vi "Teleop.vi"(10 "Match Info":T1={"Autonomous Elapsed Seconds"=0.0, "TeleOp Elapsed Seconds"=0.0, "Disabled Elapsed Seconds"=0.0, "Visited Autonomous"=FALSE, "Visited TeleOp"=FALSE, "Visited Disabled"=FALSE, "Autonomous Settings"={"Autonomous Style"=enum."Independent", "VI Refnum"=refnum}}, 11 "Call Context":T2) -> ()   [LabVIEW 2015]
doc: "This VI is called for each TeleOp packet received from the DS where the robot is not disabled. It is often used to read from the joysticks and update I/O or to update setpoints for timed control loops. It should complete and return within 20 milliseconds or it may miss DS packets."
uses:
  <vilib>/Rock Robotics/WPI/DriverStation/WPI_DriverStationDerivedRobotMode.ctl
  <vilib>/Rock Robotics/WPI/DriverStation/WPI_DriverStationMatch Info.ctl
  <vilib>/Rock Robotics/WPI/Relay/WPI_RelayValue.ctl
  <vilib>/Rock Robotics/WPI/Utilities/WPI_GetSetVariantRefNum.vi
  <vilib>/Rock Robotics/Network Tables/SD Write Boolean Array.vi
  <vilib>/Rock Robotics/Network Tables/SD Write Numeric Array.vi
  <vilib>/Rock Robotics/Network Tables/SD Read Boolean.vi
  <vilib>/Rock Robotics/Network Tables/SD Read Number.vi
  <vilib>/Rock Robotics/WPI/RobotDrive/WPI_RobotDriveMecanumDrive_Cartesian.vi
panel:
  out "Sample Slider 0":dbl(slide) scale=0.0..5.0
  out "Sample Boolean 1":bool
  out "Sample Boolean 0":bool
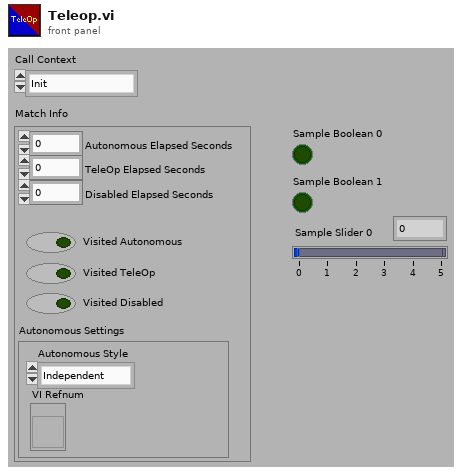
[diagram p1: front panel]
types:
  T1 = typedef "WPI_DriverStationMatch Info.ctl" = cluster{"Autonomous Elapsed Seconds":dbl, "TeleOp Elapsed Seconds":dbl, "Disabled Elapsed Seconds":dbl, "Visited Autonomous":bool, "Visited TeleOp":bool, "Visited Disabled":bool, "Autonomous Settings":cluster{"Autonomous Style":enum16{"Iterative", "Independent"}, "VI Refnum":refnum<vi>}}
  T2 = typedef "WPI_DriverStationDerivedRobotMode.ctl" = enum16{"Init", "Execute", "Stop"}
  T3 = typedef "WPI_RelayValue.ctl" = enum16{"Off", "On", "Forward", "Reverse"}
  T4 = typedef "WPI_JoystickDevRef.ctl" = cluster{"Device":T5}
  T5 = typedef "WPI_JoystickDeviceEnum.ctl" = enum16{"USB 0", "USB 1", "USB 2", "USB 3", "USB 4", "USB 5"}
  T6 = cluster{"Axes[0]":dbl, "Axes[1]":dbl, "Axes[2]":dbl, "Axes[3]":dbl, "Axes[4]":dbl, "Axes[5]":dbl, "Axes[6]":dbl, "Axes[7]":dbl, "Axes[8]":dbl}
  T7 = cluster{"Buttons[0]":bool, "Buttons[1]":bool, "Buttons[2]":bool, "Buttons[3]":bool, "Buttons[4]":bool, "Buttons[5]":bool, "Buttons[6]":bool, "Buttons[7]":bool, "Buttons[8]":bool}
  T8 = typedef "WPI_SwitchDevRef.ctl" = cluster{"DevStatus":errorcluster, "DIO Channel":T9, "CntIndex":T10, "Normally Closed":bool}
  T9 = typedef "FPGA_DIOChannel.ctl" = enum8{"DIO 0", "DIO 1", "DIO 2", "DIO 3", "DIO 4", "DIO 5", "DIO 6", "DIO 7", "DIO 8", "DIO 9", "DIO MXP 0", "DIO MXP 1", "DIO MXP 2", "DIO MXP 3", "DIO MXP 4", "DIO MXP 5", "DIO MXP 6", "DIO MXP 7", "DIO MXP 8", "DIO MXP 9", "DIO MXP 10", "DIO MXP 11", "DIO MXP 12", "DIO MXP 13", "DIO MXP 14", "DIO MXP 15", "Invalid"}
  T10 = typedef "FPGA_CounterCtrSystemIndex.ctl" = enum8{"Ctr 0", "Ctr 1", "Ctr 2", "Ctr 3", "Ctr 4", "Ctr 5", "Ctr 6", "Ctr 7", "Invalid"}
  T11 = typedef "WPI_RobotDriveDevRef.ctl" = cluster{"DevStatus":errorcluster, "Motors[]":T12[], "Square Inputs":bool, "Max Output":dbl}
  T12 = typedef "WPI_MotorControlDeviceRef.ctl" = cluster{"DeviceStatus":errorcluster, "Type":T13, "PWM":cluster{"PWM Channel":T14, "DeadBand":T15}, "CAN":cluster{"Device Number":u8, "Control Mode":T16, "Semaphore":T17, "Max Vout":dbl, "TalonSRX Control Mode":T18}, "Invert":bool}
  T13 = typedef "WPI_MotorControlType.ctl" = enum16{"PWM", "CAN", "CANTalonSRX"}
  T14 = typedef "FPGA_DIOPWMChannel.ctl" = enum8{"PWM 0", "PWM 1", "PWM 2", "PWM 3", "PWM 4", "PWM 5", "PWM 6", "PWM 7", "PWM 8", "PWM 9", "PWM MXP 0", "PWM MXP 1", "PWM MXP 2", "PWM MXP 3", "PWM MXP 4", "PWM MXP 5", "PWM MXP 6", "PWM MXP 7", "PWM MXP 8", "PWM MXP 9", "Invalid"}
  T15 = typedef "WPI_PWMDeadband.ctl" = cluster{"Name":string, "maxPositivePwm":i32, "minPositivePwm":i32, "centerPwm":i32, "maxNegativePwm":i32, "minNegativePwm":i32, "angularRange":u16}
  T16 = typedef "WPI_CANJaguar_ControlMode.ctl" = enum8{"Percent VBus", "Current", "Speed", "Position", "Voltage"}
  T17 = typedef "Semaphore RefNum" = refnum<k1>
  T18 = typedef "WPI_CANTalonSRX_APIControlMode.ctl" = enum8{"Percent VBus", "Speed", "Position", "Slave", "Unchanged / Invalid", "Voltage Compensation", "Current", "Motion Profile"}
  T19 = typedef "WPI_RelayDevRef.ctl" = cluster{"DevStatus":errorcluster, "Relay Channel":T20, "Relay Direction":T21}
  T20 = typedef "FPGA_DIORelayChannel.ctl" = enum8{"Relay 0", "Relay 1", "Relay 2", "Relay 3", "Invalid"}
  T21 = typedef "WPI_RelayDirection.ctl" = enum16{"Both directions", "Forward only", "Reverse only"}
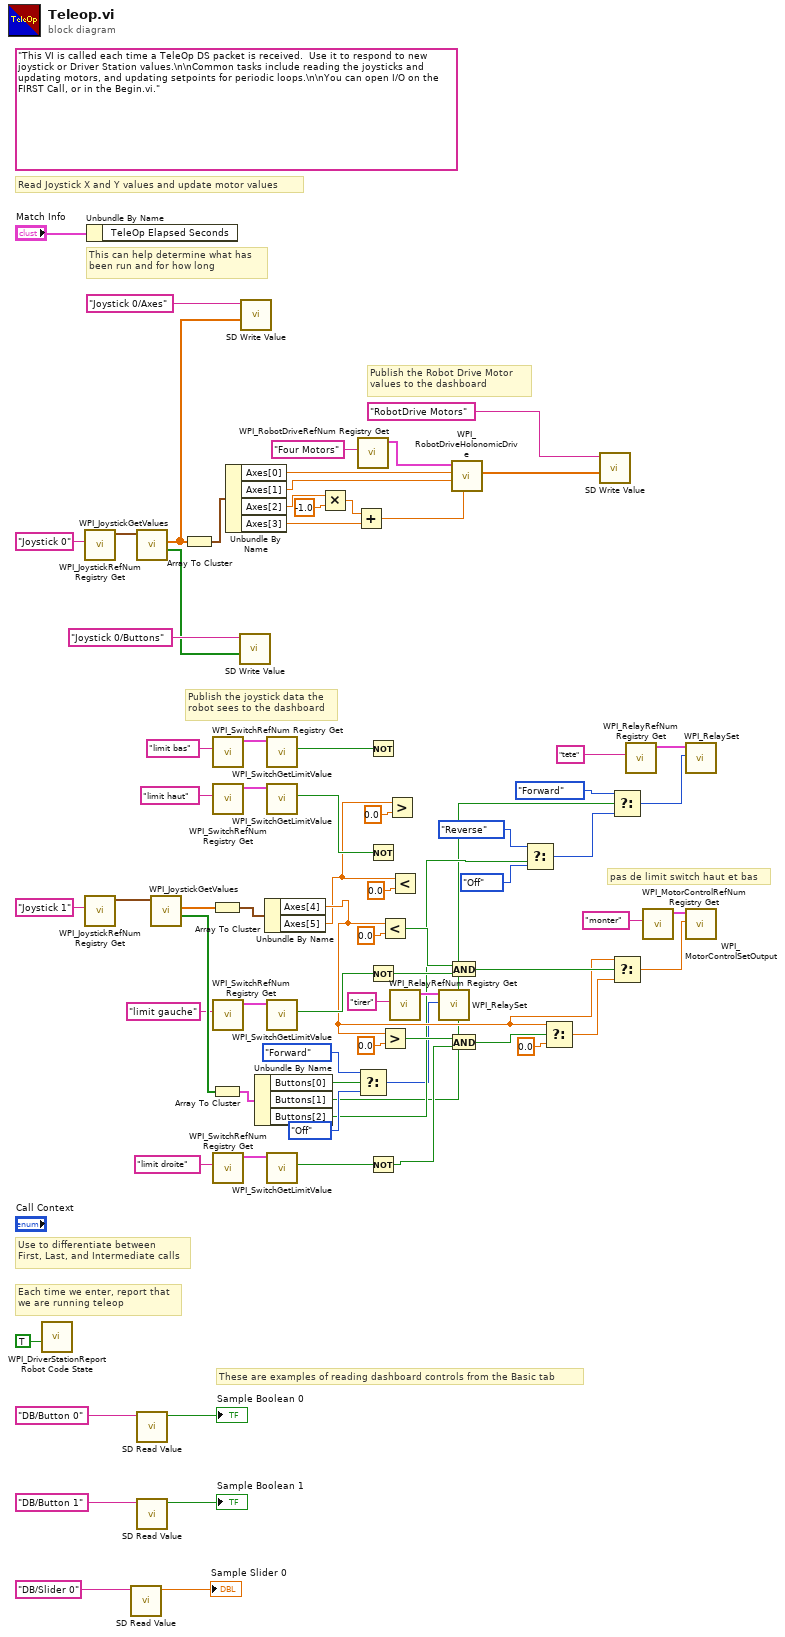
[diagram p0: block diagram]
diagram:
  (unwired) "This VI is called each time a TeleOp DS packet is received.  Use it to respond to new joystick or Driver Station values.\n\nCommon tasks include reading the joysticks and updating motors, and updating setpoints for periodic loops.\n\nYou can open I/O on the FIRST Call, or in the Begin.vi."
  # "pas de limit switch haut et bas"
  # "These are examples of reading dashboard controls from the Basic tab"
  # "Publish the Robot Drive Motor\nvalues to the dashboard"
  # "Publish the joystick data the\nrobot sees to the dashboard"
  # "Each time we enter, report that\nwe are running teleop"
  # "Use to differentiate between\nFirst, Last, and Intermediate calls"
  # "This can help determine what has\nbeen run and for how long"
  # "Read Joystick X and Y values and update motor values"
  n1 = call <vilib>:"WPI_DriverStationReport Robot Code State.vi"("TeleOp"=TRUE ("Autonomous")) -> ()  [unwired: 10 in, 1 out]
  n2 = call <vilib>:"WPI_JoystickRefNum Registry Get.vi"("refnum name"="Joystick 0") -> ("JoystickDevRef"=w72:T4)  [unwired: 1 in, 9 out]
  n3 = call <vilib>:"WPI_JoystickRefNum Registry Get.vi"("refnum name"="Joystick 1") -> ("JoystickDevRef"=w15:T4)  [unwired: 1 in, 9 out]
  n4 = Unbundle By Name("Match Info") -> ()  [unwired: 1 out]
  n5 = call-poly <vilib>:"SD Read Value.vi"("Name"="DB/Slider 0" ("refnum name")) -> ("Numeric"=→"Sample Slider 0":dbl)  [unwired: 8 in, 2 out]
  n6 = call <vilib>:"WPI_JoystickGetValues.vi"("JoystickDevRef"=w72) -> ("Buttons"=w20:bool[], "Axes"=w60:dbl[])  [unwired: 6 in, 3 out]
  n7 = call-poly <vilib>:"SD Read Value.vi"("Name"="DB/Button 0" ("refnum name")) -> ("Boolean"=→"Sample Boolean 0":bool)  [unwired: 8 in, 2 out]
  n8 = call-poly <vilib>:"SD Read Value.vi"("Name"="DB/Button 1" ("refnum name")) -> ("Boolean"=→"Sample Boolean 1":bool)  [unwired: 8 in, 2 out]
  n9 = call <vilib>:"WPI_JoystickGetValues.vi"("JoystickDevRef"=w15) -> ("Buttons"=w13:bool[], "Axes"=w12:dbl[])  [unwired: 6 in, 3 out]
  n10 = Array To Cluster(array=w60) -> (cluster=w59:T6)
  n11 = Array To Cluster(array=w12) -> (cluster=w11:T6)
  n12 = Array To Cluster(array=w13) -> (cluster=w10:T7)
  n13 = call <vilib>:"WPI_SwitchRefNum Registry Get.vi"("refnum name"="limit bas") -> ("SwitchDevRef"=w31:T8)  [unwired: 9 in, 1 out]
  n14 = call <vilib>:"WPI_SwitchRefNum Registry Get.vi"("refnum name"="limit haut") -> ("SwitchDevRef"=w33:T8)  [unwired: 9 in, 1 out]
  n15 = call <vilib>:"WPI_SwitchRefNum Registry Get.vi"("refnum name"="limit gauche") -> ("SwitchDevRef"=w47:T8)  [unwired: 9 in, 1 out]
  n16 = call <vilib>:"WPI_SwitchRefNum Registry Get.vi"("refnum name"="limit droite") -> ("SwitchDevRef"=w49:T8)  [unwired: 9 in, 1 out]
  n17 = Unbundle By Name(w59) -> ("Axes[0]"=w58:dbl, "Axes[1]"=w57:dbl, "Axes[2]"=w56:dbl, "Axes[3]"=w51:dbl)
  n18 = call-poly <vilib>:"SD Write Value.vi"("Boolean Array"=w20, "Name"="Joystick 0/Buttons") -> ()  [unwired: 8 in, 2 out]
  n19 = call-poly <vilib>:"SD Write Value.vi"("Numeric Array"=w60, "Name"="Joystick 0/Axes") -> ()  [unwired: 8 in, 2 out]
  n20 = Unbundle By Name(w10) -> ("Buttons[0]"=w9:bool, "Buttons[1]"=w3:bool, "Buttons[2]"=w5:bool)
  n21 = Unbundle By Name(w11) -> ("Axes[4]"=w7:dbl, "Axes[5]"=w6:dbl)
  n22 = call <vilib>:"WPI_SwitchGetLimitValue.vi"("SwitchDevRef"=w31) -> ("Switch Pressed"=w21:bool)  [unwired: 8 in, 2 out]
  n23 = call <vilib>:"WPI_SwitchGetLimitValue.vi"("SwitchDevRef"=w33) -> ("Switch Pressed"=w22:bool)  [unwired: 8 in, 2 out]
  n24 = call <vilib>:"WPI_SwitchGetLimitValue.vi"("SwitchDevRef"=w47) -> ("Switch Pressed"=w45:bool)  [unwired: 8 in, 2 out]
  n25 = call <vilib>:"WPI_SwitchGetLimitValue.vi"("SwitchDevRef"=w49) -> ("Switch Pressed"=w38:bool)  [unwired: 8 in, 2 out]
  n26 = Multiply(x=w56, y=-1.0) -> (x*y=w52:dbl)
  n27 = Add(x=w52, y=w51) -> (x+y=w50:dbl)
  n28 = call <vilib>:"WPI_RobotDriveRefNum Registry Get.vi"("refnum name"="Four Motors") -> ("RobotDriveDevRef"=w74:T11)  [unwired: 1 in, 9 out]
  n29 = Select(t=WPI_RelayValue."Forward", s=w9, f=WPI_RelayValue."Off" ("RelayValue")) -> (s? t:f=w1:T3)
  n30 = Not(x=w21) -> ()  [unwired: 1 out]
  n31 = Not(x=w22) -> ()  [unwired: 1 out]
  n32 = Not(x=w45) -> (.not. x?=w43:bool)
  n33 = Not(x=w38) -> (.not. x?=w4:bool)
  n34 = Less?(x=w7, y=0.0) -> (x < y?=w44:bool)
  n35 = Greater?(x=w7, y=0.0) -> (0:w40:bool)
  n36 = Greater?(x=w6, y=0.0) -> ()  [unwired: 1 out]
  n37 = Less?(x=w6, y=0.0) -> ()  [unwired: 1 out]
  n38 = call <vilib>:"WPI_RelayRefNum Registry Get.vi"("refnum name"="tirer") -> ("RelayDevRef"=w19:T19)  [unwired: 9 in, 1 out]
  n39 = call <vilib>:"WPI_RelaySet.vi"("RelayValue"=w1, "RelayDevRef"=w19) -> ()  [unwired: 8 in, 2 out]
  n40 = And(x=w44, y=w43) -> (x .and. y?=w42:bool)
  n41 = And(x=w40, y=w4) -> (x .and. y?=w2:bool)
  n42 = call-poly <vilib>:"WPI_RobotDriveHolonomicDrive.vi"("Rotation"=w50, "Y"=w57, "X"=w58, "RobotDriveDevRef"=w74) -> ("Motor Values"=w61:dbl[])  [unwired: 5 in, 2 out]
  n43 = Select(t=WPI_RelayValue."Reverse", s=w5, f=WPI_RelayValue."Off" ("RelayValue")) -> (s? t:f=w26:T3)
  n44 = Select(t=w7, s=w2, f=0.0) -> (s? t:f=w37:dbl)
  n45 = call-poly <vilib>:"SD Write Value.vi"("Numeric Array"=w61, "Name"="RobotDrive Motors") -> ()  [unwired: 8 in, 2 out]
  n46 = Select(t=WPI_RelayValue."Forward", s=w3, f=w26) -> (s? t:f=w24:T3)
  n47 = Select(t=w7, s=w42, f=w37) -> (s? t:f=w41:dbl)
  n48 = call <vilib>:"WPI_RelayRefNum Registry Get.vi"("refnum name"="tete") -> ("RelayDevRef"=w29:T19)  [unwired: 9 in, 1 out]
  n49 = call <vilib>:"WPI_MotorControlRefNum Registry Get.vi"("refnum name"="monter") -> ("MotorControlDevRef"=w54:T12)  [unwired: 9 in, 1 out]
  n50 = call <vilib>:"WPI_RelaySet.vi"("RelayValue"=w24, "RelayDevRef"=w29) -> ()  [unwired: 8 in, 2 out]
  n51 = call <vilib>:"WPI_MotorControlSetOutput.vi"("Output"=w41, "MotorControlDevRef"=w54) -> ()  [unwired: 7 in, 3 out]
